vi "NTC codes.vi"(0 "NTC Messages":T1(array[cluster])=[{"ID"=1808, "MSGTYPE"=0, "LEN"=8, "DATA[0]"=33, "DATA[1]"=11, "DATA[2]"=53, "DATA[3]"=0, "DATA[4]"=8, "DATA[5]"=0, "DATA[6]"=11, "DATA[7]"=110}, {"ID"=1808, "MSGTYPE"=0, "LEN"=8, "DATA[0]"=34, "DATA[1]"=0, "DATA[2]"=128, "DATA[3]"=0, "DATA[4]"=11, "DATA[5]"=1, "DATA[6]"=0, "DATA[7]"=131}, {"ID"=1808, "MSGTYPE"=0, "LEN"=8, "DATA[0]"=35, "DATA[1]"=0, "DATA[2]"=11, "DATA[3]"=130, "DATA[4]"=0, "DATA[5]"=133, "DATA[6]"=0, "DATA[7]"=11}, {"ID"=1808, "MSGTYPE"=0, "LEN"=8, "DATA[0]"=36, "DATA[1]"=130, "DATA[2]"=0, "DATA[3]"=140, "DATA[4]"=0, "DATA[5]"=11, "DATA[6]"=128, "DATA[7]"=0}, {"ID"=1808, "MSGTYPE"=0, "LEN"=8, "DATA[0]"=37, "DATA[1]"=142, "DATA[2]"=0, "DATA[3]"=11, "DATA[4]"=128, "DATA[5]"=0, "DATA[6]"=170, "DATA[7]"=0}, {"ID"=1808, "MSGTYPE"=0, "LEN"=8, "DATA[0]"=38, "DATA[1]"=11, "DATA[2]"=0, "DATA[3]"=0, "DATA[4]"=173, "DATA[5]"=0, "DATA[6]"=11, "DATA[7]"=0}, {"ID"=1808, "MSGTYPE"=0, "LEN"=8, "DATA[0]"=39, "DATA[1]"=0, "DATA[2]"=190, "DATA[3]"=0, "DATA[4]"=10, "DATA[5]"=16, "DATA[6]"=1, "DATA[7]"=3}, {"ID"=1808, "MSGTYPE"=0, "LEN"=8, "DATA[0]"=40, "DATA[1]"=0, "DATA[2]"=11, "DATA[3]"=1, "DATA[4]"=1, "DATA[5]"=49, "DATA[6]"=0, "DATA[7]"=11}, {"ID"=1808, "MSGTYPE"=0, "LEN"=8, "DATA[0]"=41, "DATA[1]"=0, "DATA[2]"=1, "DATA[3]"=57, "DATA[4]"=0, "DATA[5]"=11, "DATA[6]"=1, "DATA[7]"=1}, {"ID"=1808, "MSGTYPE"=0, "LEN"=8, "DATA[0]"=42, "DATA[1]"=189, "DATA[2]"=0, "DATA[3]"=11, "DATA[4]"=1, "DATA[5]"=1, "DATA[6]"=193, "DATA[7]"=0}, {"ID"=1808, "MSGTYPE"=0, "LEN"=8, "DATA[0]"=43, "DATA[1]"=11, "DATA[2]"=1, "DATA[3]"=1, "DATA[4]"=253, "DATA[5]"=0, "DATA[6]"=11, "DATA[7]"=59}, {"ID"=1808, "MSGTYPE"=0, "LEN"=8, "DATA[0]"=44, "DATA[1]"=0, "DATA[2]"=112, "DATA[3]"=1, "DATA[4]"=8, "DATA[5]"=0, "DATA[6]"=0, "DATA[7]"=172}, {"ID"=1808, "MSGTYPE"=0, "LEN"=8, "DATA[0]"=45, "DATA[1]"=1, "DATA[2]"=8, "DATA[3]"=0, "DATA[4]"=0, "DATA[5]"=176, "DATA[6]"=1, "DATA[7]"=8}, {"ID"=1808, "MSGTYPE"=0, "LEN"=8, "DATA[0]"=46, "DATA[1]"=0, "DATA[2]"=0, "DATA[3]"=177, "DATA[4]"=1, "DATA[5]"=8, "DATA[6]"=0, "DATA[7]"=0}]) -> (14 "NTC codes":string)   [LabVIEW 2023]
uses:
  <vilib>/Utility/file.llb/Write Delimited Spreadsheet (string).vi
panel:
  out "NTC Codes 1":string
  out "appended array 2":string[][](array[string])
  out "error out 2":errorcluster
  out "error out":errorcluster
  out "Combined NTC":i32[](array[numeric]) format="%.0x"
  out "appended array":i32[][](array[numeric]) format="%.0x"
  out "NTC codes1":i32[](array[numeric])
  out "Parameters":i32[](array[numeric]) format="%.0x"
  out "s":i32[](array[numeric]) format="%.0x"
  out "a":i32[](array[numeric])
  out "NTC codes0":i32[](array[numeric]) format="%.0x"
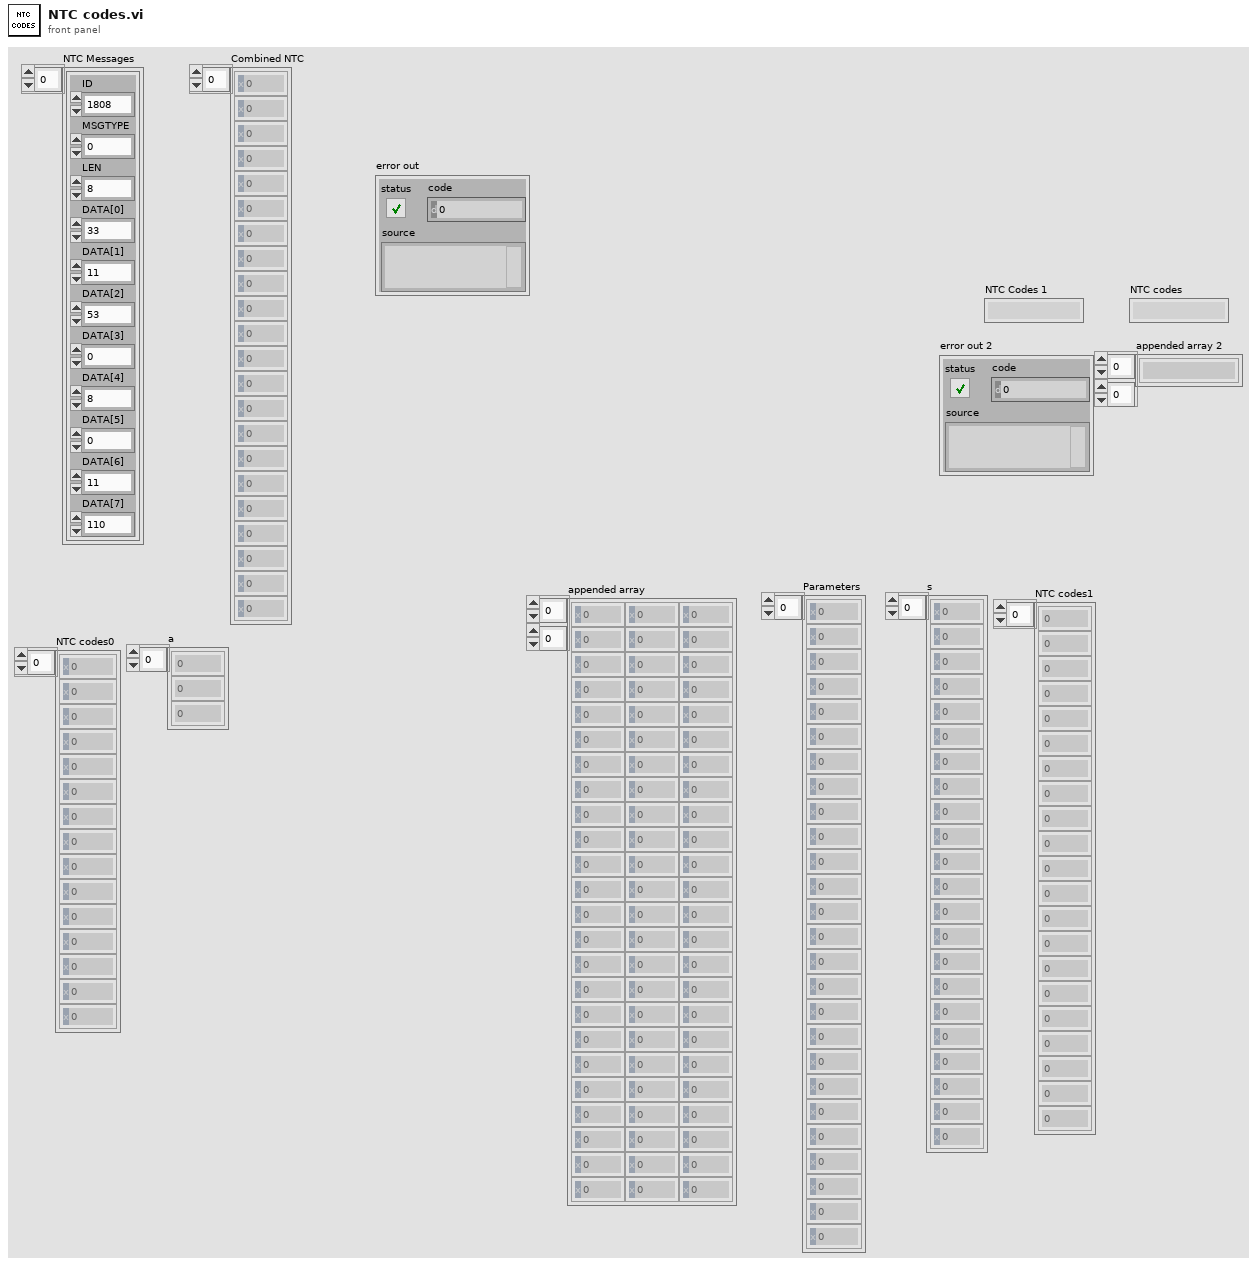
[diagram p1: front panel]
types:
  T1 = cluster{"ID":u32, "MSGTYPE":u8, "LEN":u8, "DATA[0]":u8, "DATA[1]":u8, "DATA[2]":u8, "DATA[3]":u8, "DATA[4]":u8, "DATA[5]":u8, "DATA[6]":u8, "DATA[7]":u8}[]
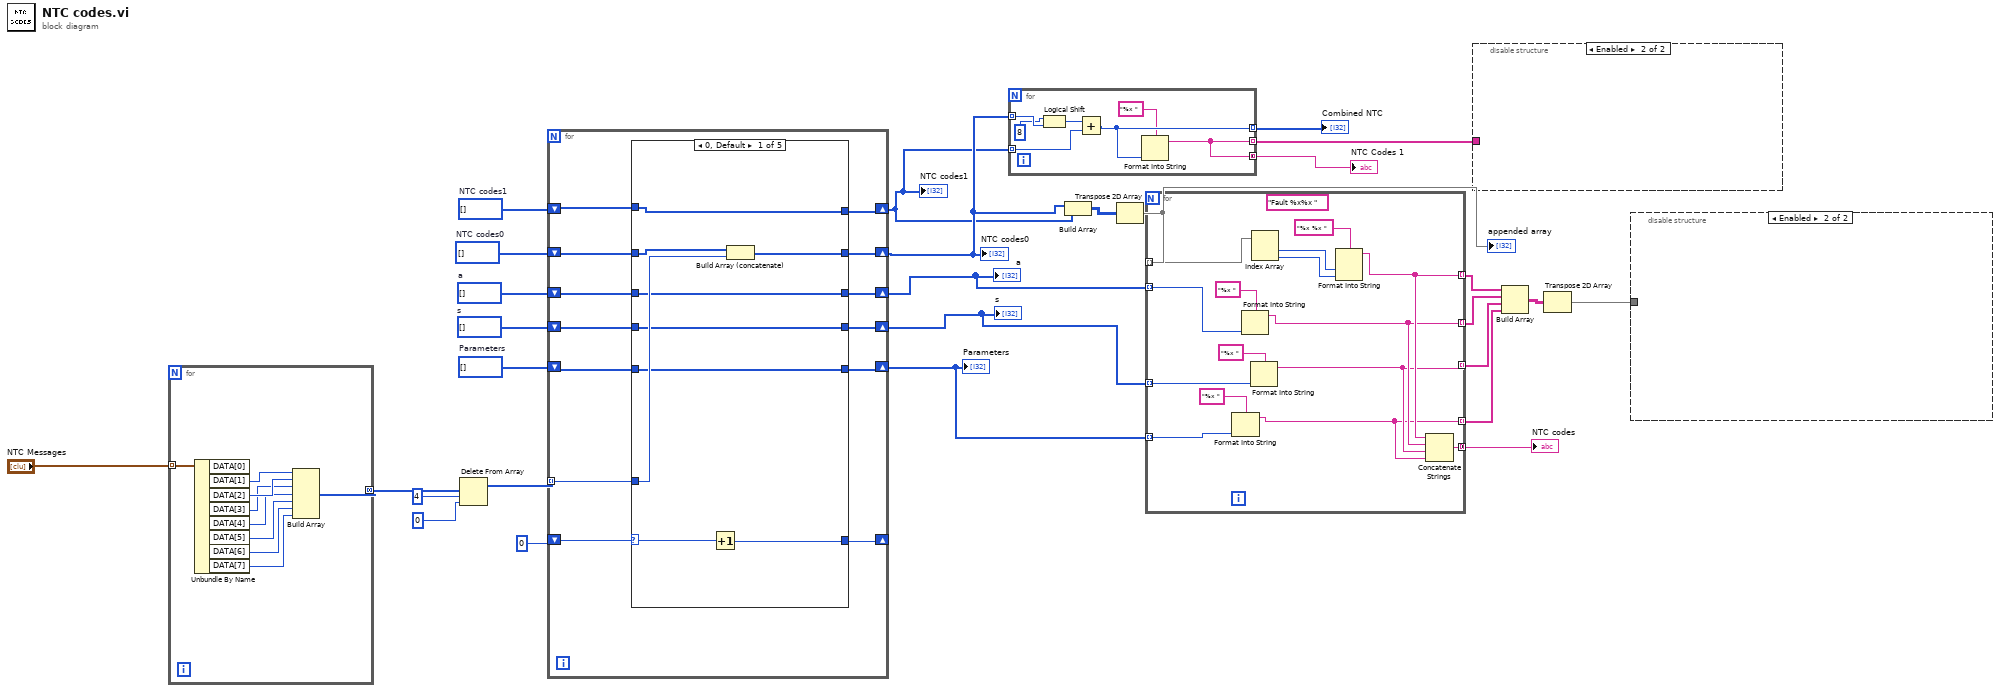
[diagram p0: block diagram]
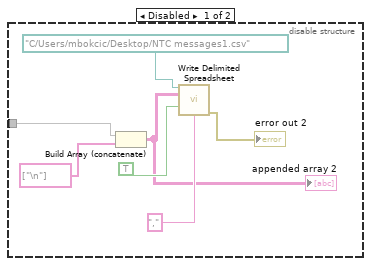
[diagram p2: hidden frame]
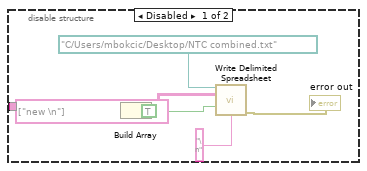
[diagram p3: hidden frame]
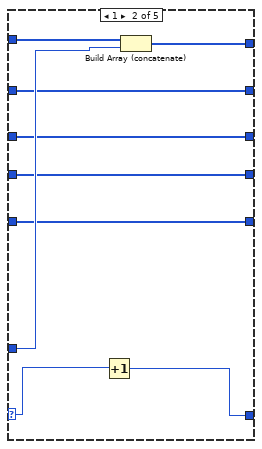
[diagram p4: hidden frame]
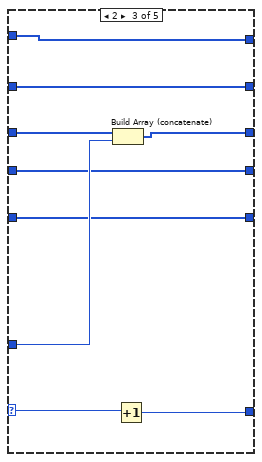
[diagram p5: hidden frame]
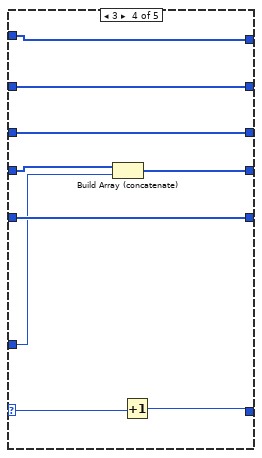
[diagram p6: hidden frame]
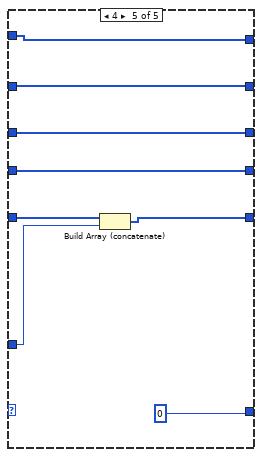
[diagram p7: hidden frame]
diagram:
  w19 = i32[] []  # NTC codes1
  w20 = i32[] []  # Parameters
  w21 = i32[] []  # s
  w22 = i32[] []  # a
  w23 = i32[] []  # NTC codes0
  n1 = for {
    tunnel: "NTC Messages" -> [w37] mode=indexing
    tunnel: [w29] -> w28 mode=concatenating
    n2 = Unbundle By Name(w37) -> ("DATA[1]"=w36:u8, "DATA[2]"=w35:u8, "DATA[3]"=w34:u8, "DATA[4]"=w33:u8, "DATA[5]"=w32:u8, "DATA[6]"=w31:u8, "DATA[7]"=w30:u8)  [unwired: 1 out]
    n3 = Build Array(w36, w35, w34, w33, w32, w31, w30) -> (w29:u8[])
  }
  n4 = Delete From Array(array=w28, length=4, index=0) -> (array with subset deleted=w25:u8[])  [unwired: 1 out]
  n5 = for {
    tunnel: w25 -> [w49] mode=indexing
    shift-right: [w40] -> _
    shift-left: 0 -> [w50]
    shift-right: [w47] -> w16
    shift-left: w23 -> [w48]
    shift-right: [w42] -> w7
    shift-left: w20 -> [w41]
    shift-right: [w43] -> w4
    shift-left: w21 -> [w44]
    shift-right: [w45] -> w9
    shift-left: w22 -> [w46]
    shift-right: [w38] -> w15
    shift-left: w19 -> [w39]
    n6 = case shown="0, Default" w50 {
      selector: w50 -> [w53 w65 w71 w80 _]
      tunnel: w49 -> [w58 w66 w74 w81 w88]
      tunnel: w48 -> [w59 w63 w77 w86 w94]
      tunnel: [w57 w63 w77 w86 w94] -> w47
      tunnel: w46 -> [w56 w62 w76 w85 w93]
      tunnel: [w56 w62 w75 w85 w93] -> w45
      tunnel: w44 -> [w55 w61 w73 w84 w92]
      tunnel: [w55 w61 w73 w83 w92] -> w43
      tunnel: [w54 w60 w72 w82 w89] -> w42
      tunnel: w41 -> [w54 w60 w72 w82 w90]
      tunnel: [w52 w64 w70 w79 0] -> w40
      tunnel: w39 -> [w51 w68 w69 w78 w87]
      tunnel: [w51 w67 w69 w78 w87] -> w38
      frame 0, Default {
        n7 = Increment(x=w53) -> (x+1=w52:i32)
        n8 = Build Array (concatenate)(w59, w58) -> (w57:i32[])
      }
      frame 1 {
        n9 = Increment(x=w65) -> (x+1=w64:i32)
        n10 = Build Array (concatenate)(w68, w66) -> (w67:i32[])
      }
      frame 2 {
        n11 = Build Array (concatenate)(w76, w74) -> (w75:i32[])
        n12 = Increment(x=w71) -> (x+1=w70:i32)
      }
      frame 3 {
        n13 = Build Array (concatenate)(w84, w81) -> (w83:i32[])
        n14 = Increment(x=w80) -> (x+1=w79:i32)
      }
      frame 4 {
        n15 = Build Array (concatenate)(w90, w88) -> (w89:i32[])
      }
    }
  }
  "NTC codes0" <- w16
  "a" <- w9
  "s" <- w4
  "Parameters" <- w7
  "NTC codes1" <- w15
  n16 = for {
    tunnel: w15 -> [w100] mode=indexing
    tunnel: w16 -> [w99] mode=indexing
    tunnel: [w97] -> w17 mode=indexing
    tunnel: [w95] -> w10 mode=indexing
    tunnel: [w95] -> w2 mode=concatenating
    n17 = Logical Shift(y=8 ("x"), x=w99) -> (x << y=w101:i32)
    n18 = Add(x=w101, y=w100) -> (x+y=w97:i32)
    n19 = Format Into String(format string="%x ", w97) -> (resulting string=w95:string)  [unwired: 2 in, 1 out]
  }
  "Combined NTC" <- w17
  "NTC Codes 1" <- w2
  n20 = Build Array(w16, w15) -> (w18:i32[][])
  n21 = Transpose 2D Array(2D array=w18) -> (transposed array=w13:i32[][])
  "appended array" <- w13
  n22 = for {
    tunnel: w13 -> [w109] mode=indexing
    tunnel: [w106] -> w12 mode=indexing
    tunnel: w9 -> [w116] mode=indexing
    tunnel: [w105] -> w8 mode=indexing
    tunnel: w7 -> [w113] mode=indexing
    tunnel: [w104] -> w6 mode=indexing
    tunnel: [w103] -> w5 mode=indexing
    tunnel: w4 -> [w112] mode=indexing
    tunnel: [w102] -> w1 mode=concatenating
    (unwired) "Fault %x%x " ("format string")
    n23 = Format Into String(format string="%x ", w113) -> (resulting string=w103:string)  [unwired: 2 in, 1 out]
    n24 = Format Into String(format string="%x ", w116) -> (resulting string=w105:string)  [unwired: 2 in, 1 out]
    n25 = Format Into String(format string="%x ", w112) -> (resulting string=w104:string)  [unwired: 2 in, 1 out]
    n26 = Index Array(array=w109) -> (element #1=w108:i32, element #2=w107:i32)  [unwired: 2 in]
    n27 = Format Into String(format string="%x %x ", w108, w107) -> (resulting string=w106:string)  [unwired: 2 in, 1 out]
    n28 = Concatenate Strings(w106, w105, w104, w103) -> (w102:string)
  }
  "NTC codes" <- w1
  n29 = disable-structure shown="Enabled" {
    disable-tunnel: w10 -> [w120 _]
    frame Disabled {
      n30 = Build Array(w120, string[] ["new \n"] ("element")) -> (w119:string[][])
      n31 = call-poly <vilib>:"Write Delimited Spreadsheet.vi"("file path (dialog if empty)"=path "C:/Users/mbokcic/Desktop/NTC combined.txt", "2D data"=w119, "append to file? (new file:F)"=TRUE, "delimiter (\\t)"="\n" ("delimiter (\\t)")) -> ("error out"=→"error out":errorcluster)  [unwired: 10 in, 1 out]
    }
    frame Enabled {
    }
  }
  n32 = Build Array(w12, w8, w6, w5) -> (w11:string[][])
  n33 = Transpose 2D Array(2D array=w11) -> (transposed array=w3:string[][])
  n34 = disable-structure shown="Enabled" {
    disable-tunnel: w3 -> [w127 _]
    frame Disabled {
      n35 = Build Array (concatenate)(w127, string[] ["\n"] ("element")) -> (w124:string[][])
      "appended array 2" <- w124
      n36 = call-poly <vilib>:"Write Delimited Spreadsheet.vi"("file path (dialog if empty)"=path "C:/Users/mbokcic/Desktop/NTC messages1.csv", "2D data"=w124, "append to file? (new file:F)"=TRUE, "delimiter (\\t)"="," ("delimiter (\\t)")) -> ("error out"=→"error out 2":errorcluster)  [unwired: 10 in, 1 out]
    }
    frame Enabled {
    }
  }
